vi "read_csv_file.vi"() -> ()   [LabVIEW 2024]
uses:
  <vilib>/Utility/file.llb/Read Delimited Spreadsheet (string).vi
panel:
  out "element":i32
  out "Array 2":i32[](array[numeric])
  out "Array":T1(array[cluster])
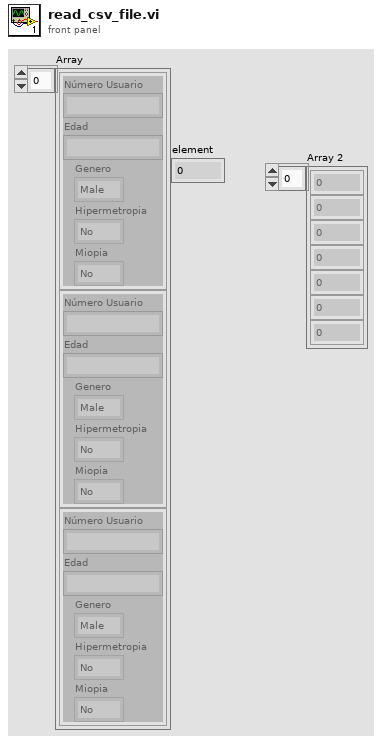
[diagram p1: front panel]
types:
  T1 = cluster{"Número Usuario":string, "Edad":string, "Genero":enum16{"Male", "Female"}, "Hipermetropia":enum16{"No", "Si"}, "Miopia":enum16{"No", "Si"}}[]
  T2 = cluster{"Número Usuario":string, "Edad":string, "Genero":enum16{"Male", "Female"}, "Hipermetropia":enum16{"No", "Si"}, "Miopia":enum16{"No", "Si"}}
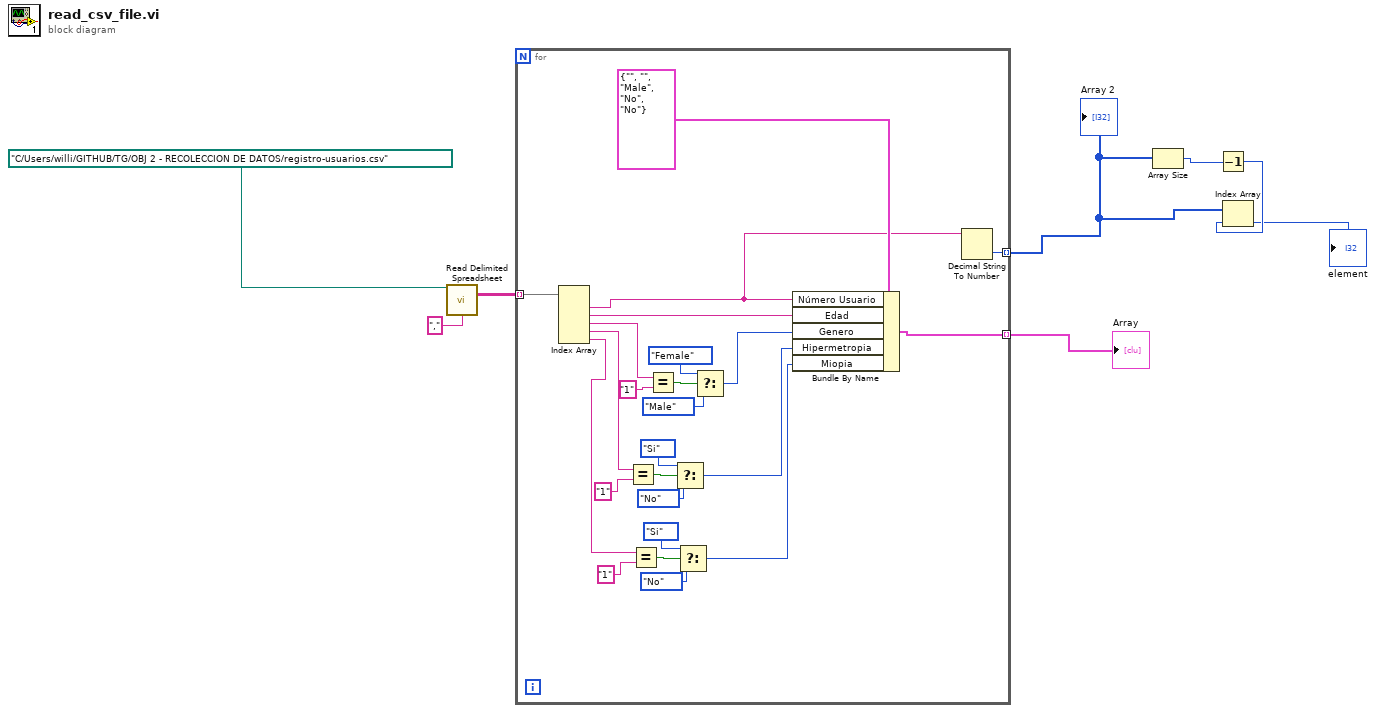
[diagram p0: block diagram]
diagram:
  n1 = call-poly <vilib>:"Read Delimited Spreadsheet.vi"("file path (dialog if empty)"=path "C:/Users/willi/GITHUB/TG/OBJ 2 - RECOLECCION DE DATOS/registro-usuarios.csv", "delimiter (\\t)"="," ("delimiter (\\t)")) -> ("all rows"=w7:string[][])  [unwired: 8 in, 5 out]
  n2 = for {
    tunnel: w7 -> [w32] mode=indexing
    tunnel: [w11] -> w6 mode=indexing
    tunnel: [w9] -> w4 mode=indexing
    n3 = Index Array(array=w32) -> (element #1=w10:string, element #2=w30:string, element #3=w28:string, element #4=w19:string, element #5=w13:string)  [unwired: 5 in]
    n4 = Equal?(x=w19, y="1") -> (x = y?=w22:bool)
    n5 = Equal?(x=w13, y="1") -> (x = y?=w16:bool)
    n6 = Equal?(x=w28, y="1") -> (x = y?=w27:bool)
    n7 = Select(t=enum16{"No", "Si"}."Si" ("Hipermetropia"), s=w22, f=enum16{"No", "Si"}."No" ("Hipermetropia")) -> (s? t:f=w18:enum16{"No", "Si"})
    n8 = Select(t=enum16{"No", "Si"}."Si" ("Hipermetropia"), s=w16, f=enum16{"No", "Si"}."No" ("Hipermetropia")) -> (s? t:f=w12:enum16{"No", "Si"})
    n9 = Select(t=enum16{"Male", "Female"}."Female" ("Genero"), s=w27, f=enum16{"Male", "Female"}."Male" ("Genero")) -> (s? t:f=w24:enum16{"Male", "Female"})
    n10 = Bundle By Name(cluster=T2 {"Número Usuario"="", "Edad"="", "Genero"=enum."Male", "Hipermetropia"=enum."No", "Miopia"=enum."No"} ("Registrar Usuario"), "Número Usuario"=w10, "Edad"=w30, "Genero"=w24, "Hipermetropia"=w18, "Miopia"=w12) -> (w11:T2)
    n11 = Decimal String To Number(string=w10) -> (number=w9:i32)  [unwired: 2 in, 1 out]
  }
  "Array" <- w6
  "Array 2" <- w4
  n12 = Array Size(array=w4) -> (size(s)=w3:i32)
  n13 = Decrement(x=w3) -> (x-1=w2:i32)
  n14 = Index Array(array=w4, index=w2) -> (element=→"element":i32)
